vi "TotalHits.vi"(10 "Number (0)":u64, 11 "Action":T1(ring)) -> (2 "Result":u64)   [LabVIEW 2016]
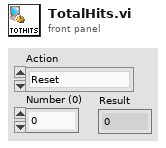
[diagram p1: front panel]
types:
  T1 = enum16{"Reset", "ReadAndReset", "Read", "Add", "Init"}
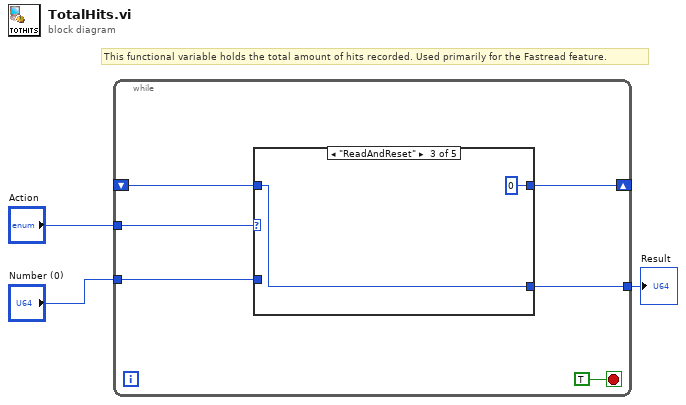
[diagram p0: block diagram]
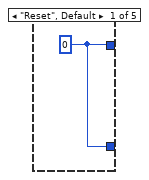
[diagram p2: hidden frame]
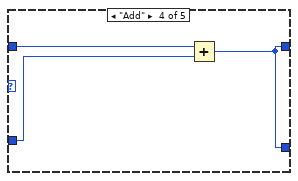
[diagram p4: hidden frame]
diagram:
  # "This functional variable holds the total amount of hits recorded. Used primarily for the Fastread feature."
  n1 = while {
    shift-right: [w5] -> _
    shift-left: _ -> [w8]
    tunnel: "Action" -> [w7]
    tunnel: "Number (0)" -> [w6]
    tunnel: [w4] -> w1
    stop <- TRUE stop-if-true
    n2 = case shown="\"ReadAndReset\"" w7 {
      tunnel: w8 -> [_ w11 w13 w16 _]
      tunnel: [w10 w11 u64 0 ("Number (0)") w14 w17] -> w5
      tunnel: w6 -> [_ _ _ w15 w17]
      tunnel: [w10 w11 w13 w14 w17] -> w4
      frame "Reset", Default {
        w10 = u64 0
      }
      frame "Read" {
      }
      frame "ReadAndReset" {
      }
      frame "Add" {
        n3 = Add(x=w16, y=w15) -> (x+y=w14:u64)
      }
      frame "Init" {
      }
    }
  }
  "Result" <- w1
